vi "Check Record Params.vi"() -> ()   [LabVIEW 2011]
uses:
  <vilib>/Utility/error.llb/DialogType.ctl
panel:
  out "error out":errorcluster
  in  "Record Length":u16=30
  in  "% of Pre-Trigger Samples":dbl=10.0
  in  "% of Hold Off Time":dbl=10.0
  in  "Record Count":u16=1
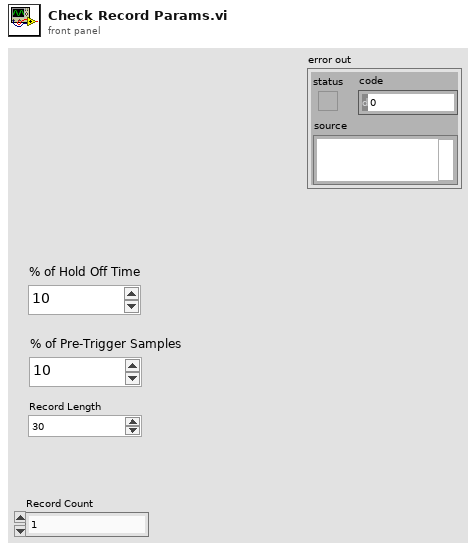
[diagram p1: front panel]
types:
  T1 = typedef "DialogType.ctl" = u16
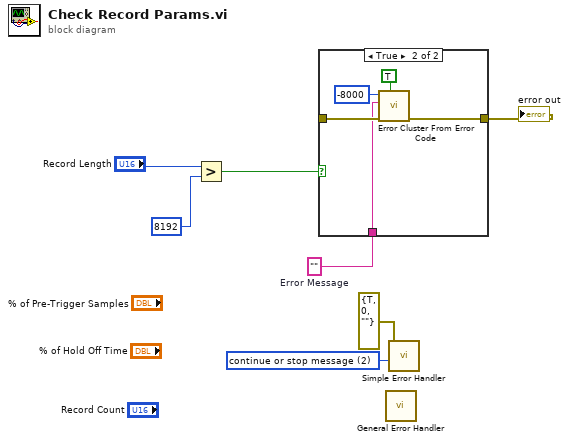
[diagram p0: block diagram]
diagram:
  w2 = T1 2 items=["no dialog", "OK message", "continue or stop message", "OK message + warnings", "continue/stop + warnings"] ("type of dialog (OK msg:1)")
  w4 = ""  # Error Message
  n1 = Greater?(x="Record Length", y=u16 8192) -> (0:w3:bool)
  n2 = case shown="True" w3 {
    tunnel: _ -> [w8 w12]
    tunnel: [w8 w11] -> w5
    tunnel: w4 -> [_ w10]
    frame False {
    }
    frame True {
      n3 = call <vilib>:"Error Cluster From Error Code.vi"("show call chain? (False)"=TRUE, "error in (no error)"=w12, "error message (\"\")"=w10, "error code (0)"=-8000) -> ("error out"=w11:errorcluster)  [unwired: 5 in]
    }
  }
  "error out" <- w5
  n4 = call <vilib>:"General Error Handler.vi"() -> ()  [unwired: 11 in, 5 out]
  n5 = call <vilib>:"Simple Error Handler.vi"("type of dialog (OK msg:1)"=w2, "error in (no error)"=errorcluster {"status"=TRUE, "code"=0, "source"=""}) -> ()  [unwired: 3 in, 5 out]
